vi "Set Mouse Icon.vi"(8 "error in (no error)":errorcluster, 10 "icon":u16, 11 "Xinformation In":T1) -> (0 "error out":errorcluster, 3 "Xinformation Out":T1)   [LabVIEW 2017, in "XGrapher.xctl"]
doc: "Sets the mouse cursor to the [index] value. Set cursor to 0 to let labview handle default cursor icon"
uses:
  XGrapher.xctl
  Typedefs/Xinformation.ctl
  Typedefs/Xcrtl-Click Operation.ctl
  <vilib>/Utility/cursorutil.llb/Set Cursor (Icon Pict).vi
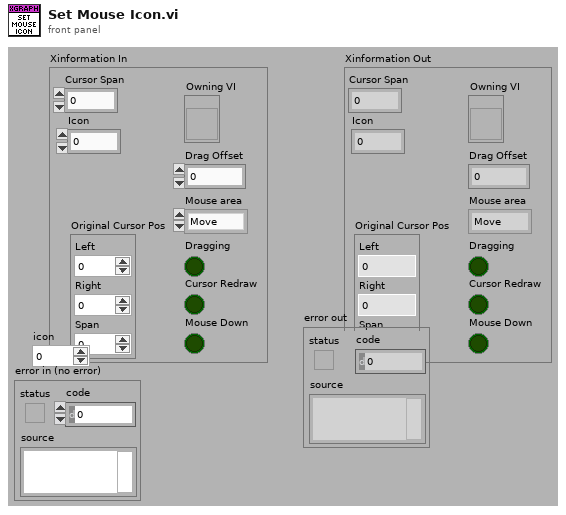
[diagram p1: front panel]
types:
  T1 = typedef "XGrapher.xctl/Xinformation.ctl" = cluster{"Cursor Span":dbl, "Icon":u16, "Mouse Down":bool, "Owning VI":refnum<vi>, "Mouse area":T2, "Dragging":bool, "Drag Offset":dbl, "Original Cursor Pos":cluster{"Left":dbl, "Right":dbl, "Span":dbl}, "Cursor Redraw":bool}
  T2 = typedef "XGrapher.xctl/Xcrtl-Click Operation.ctl" = enum16{"Move", "left cursor", "right cursor", "none"}
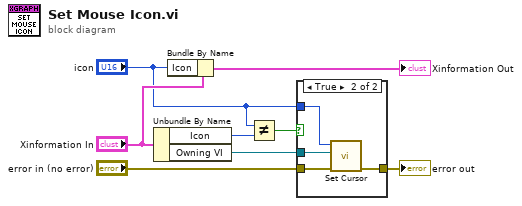
[diagram p0: block diagram]
diagram:
  n1 = Unbundle By Name("Xinformation In") -> ("Icon"=w2:u16, "Owning VI"=w3:refnum<vi>)
  n2 = Bundle By Name(cluster="Xinformation In", "Icon"="icon") -> (→"Xinformation Out":T1)
  n3 = Not Equal?(x="icon", y=w2) -> (x != y?=w7:bool)
  n4 = case shown="True" w7 {
    tunnel: "icon" -> [_ w13]
    tunnel: w3 -> [_ w12]
    tunnel: "error in (no error)" -> [w9 w11]
    tunnel: [w9 w10] -> w5
    frame False {
    }
    frame True {
      n5 = call-poly <vilib>:"Set Cursor.vi"("error in (no error)"=w11, "VI reference (current VI)"=w12, "icon"=w13) -> ("error out"=w10:errorcluster)  [unwired: 7 in, 1 out]
    }
  }
  "error out" <- w5
